vi "11-2 Noise visa.vi"() -> ()   [LabVIEW 2012]
doc: "This example demonstrates how to use the various statistics VI's in the Analysis Library to generate common descriptive statistics quantities."
uses:
  <vilib>/Analysis/baseanly.llb/Unimode.vi
  <vilib>/Analysis/NI_AALPro.lvlib
  <vilib>/Analysis/NI_AALBase.lvlib
panel:
  in  "Boolean":bool
  in  "medie":i32=9
  out "Noise 2":dbl[](graph)
  out "Histogram 2":T1(graph)
  out "Mean 2":dbl=0.028574228286743178 format="%.2f"
  out "STD 2":dbl=0.9724758954834173 format="%.2f"
  out "Variance 2":dbl=0.028574228286743168 format="%.2f"
  out "Skewness 2":dbl=0.2146149630445097 format="%.2f"
  out "Kurtosis 2":dbl=2.530711352055369 format="%.2f"
  out "Mode 2":dbl=0.23823547363281233 format="%.2f"
  out "Mode":dbl=0.23823547363281233 format="%.2f"
  out "Kurtosis":dbl=2.530711352055369 format="%.2f"
  out "Skewness":dbl=0.2146149630445097 format="%.2f"
  out "Variance":dbl=0.028574228286743168 format="%.2f"
  out "STD":dbl=0.9724758954834173 format="%.2f"
  out "Mean":dbl=0.028574228286743178 format="%.2f"
  in  "Intervals":i32=100
  in  "Samples":i32=500
  out "Noise":dbl[](graph)
  out "Histogram":T1(graph)
  # "Modificare  il VI NoiseExample in modo da visualizzare il rumore prodotto dal Generatore HP33120A ed acquisito dal multimetro HP34401A\n(utilizzare i VI Hp34401-n-meas e  hp33120a-Wfm config ex"
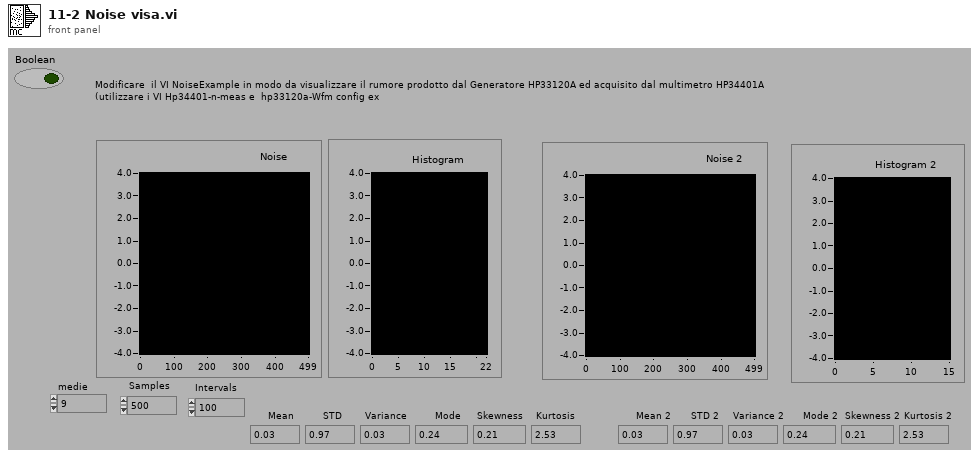
[diagram p1: front panel]
types:
  T1 = cluster{"Histogram: h(x)":i32[], "X Values":dbl[]}
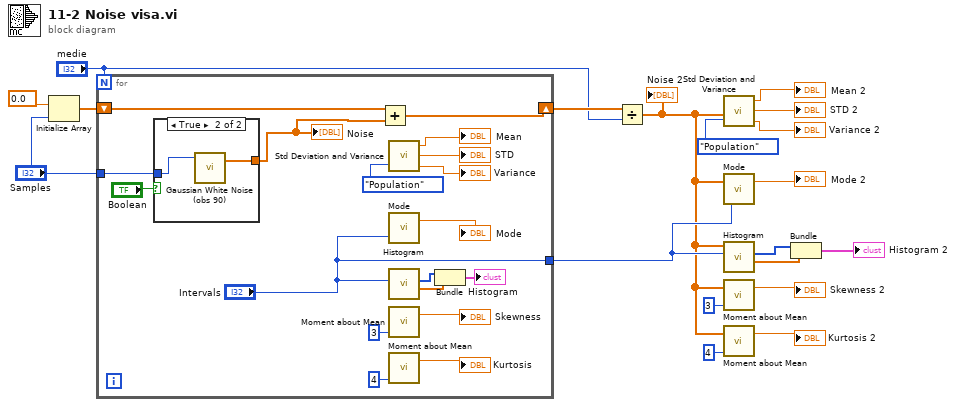
[diagram p0: block diagram]
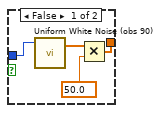
[diagram p2: hidden frame]
diagram:
  n1 = Initialize Array(0.0 ("Element Data"), "Samples") -> (w1:dbl[])
  n2 = for {
    N: "medie" -> [_]
    tunnel: ["Intervals"] -> w7
    shift-right: [w24] -> w6
    shift-left: w1 -> [w23]
    tunnel: "Samples" -> [w21]
    n3 = case shown="True" "Boolean" {
      tunnel: w21 -> [w41 w43]
      tunnel: [w38 w42] -> w20
      frame False {
        n4 = call <vilib>:"Uniform White Noise (obs 90).vi"("samples"=w41) -> ("uniform white noise"=w39:dbl[])  [unwired: 2 in, 1 out]
        n5 = Multiply(x=w39, y=50.0) -> (x*y=w38:dbl[])
      }
      frame True {
        n6 = call <vilib>:"Gaussian White Noise (obs 90).vi"("samples"=w43) -> ("Gaussian noise pattern"=w42:dbl[])  [unwired: 2 in, 1 out]
      }
    }
    "Noise" <- w20
    n7 = Add(x=w23, y=w20) -> (x+y=w24:dbl[])
    n8 = call <vilib>:"Std Deviation and Variance.vi"("Weighting (Sample)"=enum16{"Sample", "Population"}."Population") -> ("mean"=→"Mean":dbl, "standard deviation"=→"STD":dbl, "variance"=→"Variance":dbl)  [unwired: 1 in]
    n9 = call-poly <vilib>:"Mode.vi"("intervals"="Intervals") -> ("mode"=→"Mode":dbl)  [unwired: 1 in, 1 out]
    n10 = call <vilib>:"Histogram.vi"("intervals"="Intervals") -> ("X Values"=w37:dbl[], "Histogram: h(x)"=w36:i32[])  [unwired: 7 in, 2 out]
    n11 = call <vilib>:"Moment about Mean.vi"("order"=3) -> ("moment"=→"Skewness":dbl)  [unwired: 1 in, 1 out]
    n12 = call <vilib>:"Moment about Mean.vi"("order"=4) -> ("moment"=→"Kurtosis":dbl)  [unwired: 1 in, 1 out]
    n13 = Bundle("Histogram: h(x)"=w36, "X Values"=w37) -> (→"Histogram":T1)  [unwired: 1 in]
  }
  n14 = Divide(x=w6, y="medie") -> (x/y=w4:dbl[])
  "Noise 2" <- w4
  n15 = call <vilib>:"Std Deviation and Variance.vi"("X"=w4, "Weighting (Sample)"=enum16{"Sample", "Population"}."Population") -> ("mean"=→"Mean 2":dbl, "standard deviation"=→"STD 2":dbl, "variance"=→"Variance 2":dbl)
  n16 = call-poly <vilib>:"Mode.vi"("intervals"=w7, "X"=w4) -> ("mode"=→"Mode 2":dbl)  [unwired: 1 out]
  n17 = call <vilib>:"Histogram.vi"("intervals"=w7, "X"=w4) -> ("X Values"=w8:dbl[], "Histogram: h(x)"=w9:i32[])  [unwired: 6 in, 2 out]
  n18 = call <vilib>:"Moment about Mean.vi"("order"=3, "X"=w4) -> ("moment"=→"Skewness 2":dbl)  [unwired: 1 out]
  n19 = call <vilib>:"Moment about Mean.vi"("order"=4, "X"=w4) -> ("moment"=→"Kurtosis 2":dbl)  [unwired: 1 out]
  n20 = Bundle("Histogram: h(x)"=w9, "X Values"=w8) -> (→"Histogram 2":T1)  [unwired: 1 in]
